vi "WPI_UtilitiesFRCAutomaticValuePublisherImpl.vi"(11 "Enable":bool=TRUE) -> ()   [LabVIEW 2017]
uses:
  <vilib>/Rock Robotics/WPI/Utilities/Refnum Registry Operation.ctl
  <vilib>/Rock Robotics/WPI/Ultrasonic/WPI_SonarSRF04DigitalRefNum Registry Get.vi
  <vilib>/Rock Robotics/WPI/Ultrasonic/WPI_SonarSRF04DigitalGetRange.vi
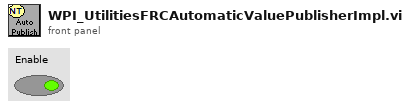
[diagram p1: front panel]
types:
  T1 = typedef "Refnum Registry Operation.ctl" = enum16{"set", "get", "delete", "get all names", "read name"}
  T2 = typedef "WPI_JoystickDevRef.ctl" = cluster{"Device":T3}
  T3 = typedef "WPI_JoystickDeviceEnum.ctl" = enum16{"USB 0", "USB 1", "USB 2", "USB 3", "USB 4", "USB 5"}
  T4 = typedef "WPI_Joystick Info.ctl" = cluster{"Device Name":string, "HID Type":T5, "XBox Type":T6, "Axes Count":i32, "Axes Types":T7[], "Button Count":i32, "POV Count":i32}
  T5 = typedef "WPI_JoystickHID Types.ctl" = enum16{"Not HID", "HID Joystick", "HID Gamepad", "HID Driving Wheel", "HID Flightstick", "HID First Person"}
  T6 = typedef "WPI_JoystickXBox Types.ctl" = enum16{"Not XBox", "XBox Unknown", "XBox Gamepad", "XBox Wheel", "XBox Arcade Stick", "XBox Flight Stick", "XBox Dance Pad", "XBox Guitar", "XBox Drum Kit", "XBox Arcade Pad"}
  T7 = typedef "WPI_JoystickAxis Types.ctl" = enum16{"X Axis", "Y Axis", "Z Axis", "RxAxis", "RyAxis", "RzAxis", "Slider", "POV", "None", "L X Axis", "L Y Axis", "L Trigger", "R Trigger", "R X Axis", "R Y Axis"}
  T8 = typedef "WPI_MotorControlDeviceRef.ctl" = cluster{"DeviceStatus":errorcluster, "Type":T9, "PWM":cluster{"PWM Channel":T10, "DeadBand":T11}, "CAN":cluster{"Device Number":u8, "SetOutput VI Ref":variant, "GetOutput VI Ref":variant, "Enable VI Ref":variant, "Disable VI Ref":variant, "Data":variant}, "Invert":bool, "DIO PWM":cluster{"PWM \"Enable\" Channel":T10, "DIOChannel":T12, "PWM Rate":dbl}}
  T9 = typedef "WPI_MotorControlType.ctl" = enum16{"PWM", "CAN", "DIO PWM"}
  T10 = typedef "FPGA_DIOPWMChannel.ctl" = enum8{"PWM 0", "PWM 1", "PWM 2", "PWM 3", "PWM 4", "PWM 5", "PWM 6", "PWM 7", "PWM 8", "PWM 9", "PWM MXP 0", "PWM MXP 1", "PWM MXP 2", "PWM MXP 3", "PWM MXP 4", "PWM MXP 5", "PWM MXP 6", "PWM MXP 7", "PWM MXP 8", "PWM MXP 9", "Invalid"}
  T11 = typedef "WPI_PWMDeadband.ctl" = cluster{"Name":string, "maxPositivePwm":i32, "minPositivePwm":i32, "centerPwm":i32, "maxNegativePwm":i32, "minNegativePwm":i32, "angularRange":u16}
  T12 = typedef "FPGA_DIOChannel.ctl" = enum8{"DIO 0", "DIO 1", "DIO 2", "DIO 3", "DIO 4", "DIO 5", "DIO 6", "DIO 7", "DIO 8", "DIO 9", "DIO MXP 0", "DIO MXP 1", "DIO MXP 2", "DIO MXP 3", "DIO MXP 4", "DIO MXP 5", "DIO MXP 6", "DIO MXP 7", "DIO MXP 8", "DIO MXP 9", "DIO MXP 10", "DIO MXP 11", "DIO MXP 12", "DIO MXP 13", "DIO MXP 14", "DIO MXP 15", "SPI Port CS1", "SPI Port CS2", "SPI Port CS3", "SPI Port MISO", "SPI Port MOSI", "Invalid"}
  T13 = typedef "WPI_ServoDeviceRef.ctl" = cluster{"DeviceStatus":errorcluster, "PWM Channel":T10, "DeadBand":T11}
  T14 = typedef "WPI_GyroDevRef.ctl" = cluster{"DevStatus":errorcluster, "Analog Channel":T15, "Gain (VoltsPerDegree/Second)":dbl, "Gyro Type":enum16{"Analog", "XRS450"}, "Handle":i32, "SPI Bus":T16, "Device Found":bool, "Sample Rate":dbl, "Calibrate On Open":bool, "Offset":dbl}
  T15 = typedef "FPGA_AIChannel.ctl" = enum8{"AI 0", "AI 1", "AI 2", "AI 3", "AI MXP 0", "AI MXP 1", "AI MXP 2", "AI MXP 3", "Invalid"}
  T16 = typedef "spi_bus.ctl" = enum16{"SPI On-Board, CS0", "SPI On-Board, CS1", "SPI On-Board, CS2", "SPI On-Board, CS3", "SPI MXP", "Invalid"}
  T17 = typedef "WPI_UltrasonicDeviceRef.ctl" = cluster{"DevStatus":errorcluster, "Ping Channel":T12, "Echo Channel":T12, "CntIndex":T18}
  T18 = typedef "FPGA_CounterCtrSystemIndex.ctl" = enum8{"Ctr 0", "Ctr 1", "Ctr 2", "Ctr 3", "Ctr 4", "Ctr 5", "Ctr 6", "Ctr 7", "Invalid"}
  T19 = typedef "WPI_EncoderDevRef.ctl" = cluster{"DevStatus":errorcluster, "EncoderIndex":T20, "CounterIndex":T18, "DistancePerCount":dbl, "Decoding Type":T21}
  T20 = typedef "FPGA_EncoderIdx.ctl" = enum8{"Enc 0", "Enc 1", "Enc 2", "Enc 3", "Enc 4", "Enc 5", "Enc 6", "Enc 7", "Invalid"}
  T21 = typedef "WPI_EncoderType.ctl" = enum16{"1x", "2x", "4x"}
  T22 = typedef "WPI_CameraDevRef.ctl" = cluster{"Camera Address":string, "CameraStatus":errorcluster}
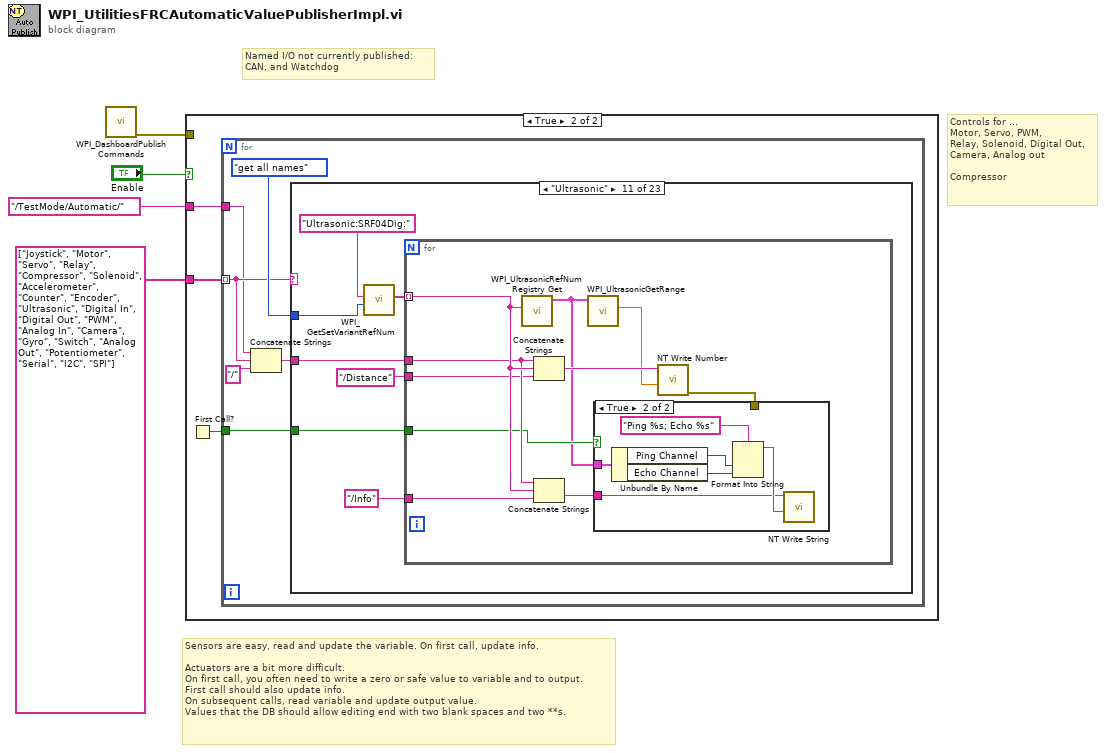
[diagram p0: block diagram]
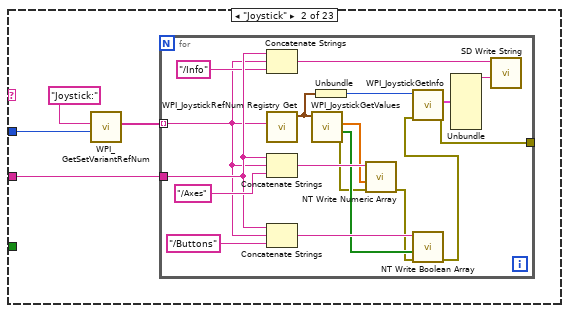
[diagram p4: hidden frame]
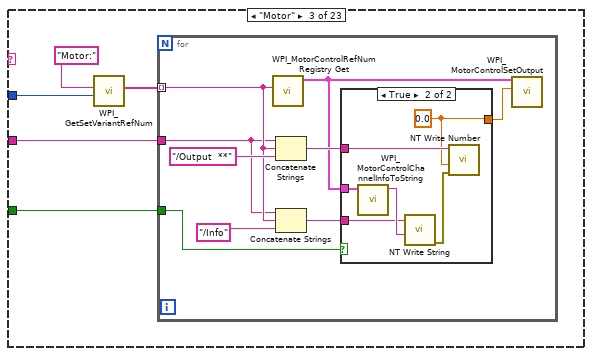
[diagram p5: hidden frame]
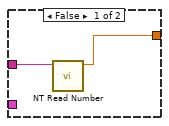
[diagram p6: hidden frame]
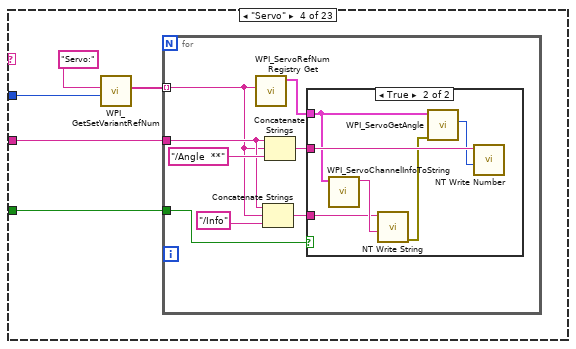
[diagram p7: hidden frame]
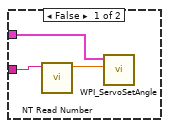
[diagram p8: hidden frame]
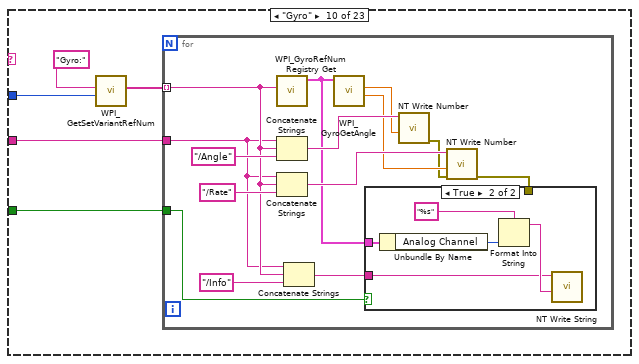
[diagram p14: hidden frame]
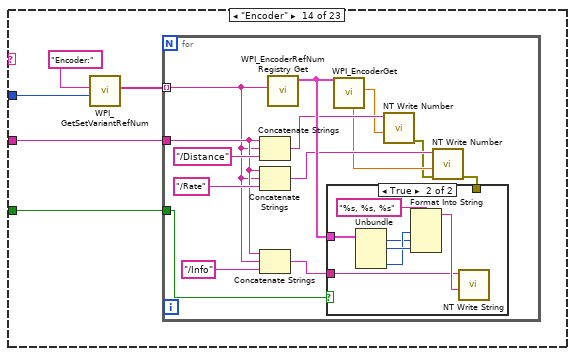
[diagram p19: hidden frame]
diagram:
  # "Controls for ...\nMotor, Servo, PWM,\nRelay, Solenoid, Digital Out,\nCamera, Analog out\n\nCompressor"
  # "Named I/O not currently published:\nCAN, and Watchdog"
  # "Sensors are easy, read and update the variable. On first call, update info.\n\nActuators are a bit more difficult. \nOn first call, you often need to write a zero or safe value to variable and to output.\nFirst call should also update info.\nOn subsequent calls, read variable and update output value.\nValues that the DB should allow editing end with two blank spaces and two **s."
  n1 = call <vilib>:"WPI_DashboardPublish Commands.vi"() -> ("error out"=w1:errorcluster)  [unwired: 11 in]
  n2 = case shown="True" "Enable" {
    tunnel: string[] ["Joystick", "Motor", "Servo", "Relay", "Compressor", "Solenoid", "Accelerometer", "Counter", "Encoder", "Ultrasonic", "Digital In", "Digital Out", "PWM", "Analog In", "Camera", "Gyro", "Switch", "Analog Out", "Potentiometer", "Serial", "I2C", "SPI"] -> [_ w7]
    tunnel: "/TestMode/Automatic/" -> [_ w5]
    tunnel: w1 -> [_ _]
    frame False {
    }
    frame True {
      n3 = First Call?() -> (First Call?: T/F=w6:bool)
      n4 = for {
        tunnel: w7 -> [w11] mode=indexing
        tunnel: w6 -> [w12]
        tunnel: w5 -> [w10]
        n5 = Concatenate Strings(w10, w11, "/") -> (w8:string)
        n6 = case shown="\"Ultrasonic\"" w11 {
          tunnel: Refnum_Registry_Operation."get all names" ("menu") -> [_ w15 w37 w58 _ _ _ _ _ w80 w108 _ _ w127 _ _ _ _ _ w153 _ _ _]
          tunnel: w12 -> [_ _ w40 w62 _ _ _ _ _ w84 w110 _ _ w131 _ _ _ _ _ w157 _ _ _]
          tunnel: w8 -> [_ w17 w39 w61 _ _ _ _ _ w83 w109 _ _ w130 _ _ _ _ _ w156 _ _ _]
          frame Default {
            # "Unsupported I/O type"
          }
          frame "Joystick" {
            n7 = call <vilib>:"WPI_GetSetVariantRefNum.vi"("Operation"=w15, "refnum name"="Joystick:") -> ("names"=w16:string[])  [unwired: 7 in, 2 out]
            n8 = for {
              tunnel: w16 -> [w24] mode=indexing
              tunnel: w17 -> [w26]
              tunnel: [w18] -> _
              n9 = Concatenate Strings(w26, w24, "/Info") -> (w23:string)
              n10 = call <vilib>:"WPI_JoystickRefNum Registry Get.vi"("refnum name"=w24) -> ("JoystickDevRef"=w29:T2)  [unwired: 9 in, 1 out]
              n11 = Concatenate Strings(w26, w24, "/Axes") -> (w32:string)
              n12 = Concatenate Strings(w26, w24, "/Buttons") -> (w34:string)
              n13 = call <vilib>:"WPI_JoystickGetValues.vi"("JoystickDevRef"=w29) -> ("error out"=w19:errorcluster, "Buttons"=w30:bool[], "Axes"=w31:dbl[])  [unwired: 6 in, 2 out]
              n14 = Unbundle(w29) -> ("Device"=w28:T3)
              n15 = call <vilib>:"NT Write Numeric Array.vi"("error in"=w19, "Numeric Array"=w31, "Name"=w32) -> ("error out"=w21:errorcluster)  [unwired: 8 in]
              n16 = call <vilib>:"NT Write Boolean Array.vi"("error in"=w21, "Boolean Array"=w30, "Name"=w34) -> ("error out"=w20:errorcluster)  [unwired: 8 in]
              n17 = call <vilib>:"WPI_JoystickGetInfo.vi"("error in (no error)"=w20, "JoystickDevice"=w28) -> ("error out"=w18:errorcluster, "Joystick Info"=w27:T4)  [unwired: 8 in]
              n18 = Unbundle(w27) -> ("Device Name"=w22:string)  [unwired: 6 out]
              n19 = call <vilib>:"SD Write String.vi"("String"=w22, "Name"=w23) -> ()  [unwired: 8 in, 2 out]
            }
          }
          frame "Motor" {
            n20 = call <vilib>:"WPI_GetSetVariantRefNum.vi"("Operation"=w37, "refnum name"="Motor:") -> ("names"=w36:string[])  [unwired: 7 in, 2 out]
            n21 = for {
              tunnel: w36 -> [w44] mode=indexing
              tunnel: w40 -> [w46]
              tunnel: w39 -> [w43]
              n22 = call <vilib>:"WPI_MotorControlRefNum Registry Get.vi"("refnum name"=w44) -> ("MotorControlDevRef"=w42:T8)  [unwired: 9 in, 1 out]
              n23 = Concatenate Strings(w43, w44, "/Output  **") -> (w48:string)
              n24 = Concatenate Strings(w43, w44, "/Info") -> (w41:string)
              n25 = case shown="True" w46 {
                tunnel: w48 -> [w51 w57]
                tunnel: [w50 w56] -> w47
                tunnel: w42 -> [_ w54]
                tunnel: w41 -> [_ w53]
                frame False {
                  n26 = call <vilib>:"NT Read Number.vi"("Name"=w51) -> ("Numeric"=w50:dbl)  [unwired: 9 in, 1 out]
                }
                frame True {
                  w56 = 0.0
                  n27 = call <vilib>:"WPI_MotorControlChannelInfoToString.vi"("MotorControlDevRef"=w54) -> ("String"=w55:string)  [unwired: 10 in]
                  n28 = call <vilib>:"NT Write String.vi"("String"=w55, "Name"=w53) -> ("error out"=w52:errorcluster)  [unwired: 9 in]
                  n29 = call <vilib>:"NT Write Number.vi"("error in"=w52, "Numeric"=w56, "Name"=w57) -> ()  [unwired: 8 in, 1 out]
                }
              }
              n30 = call <vilib>:"WPI_MotorControlSetOutput.vi"("Output"=w47, "MotorControlDevRef"=w42) -> ()  [unwired: 7 in, 3 out]
            }
          }
          frame "Servo" {
            n31 = call <vilib>:"WPI_GetSetVariantRefNum.vi"("Operation"=w58, "refnum name"="Servo:") -> ("names"=w59:string[])  [unwired: 7 in, 2 out]
            n32 = for {
              tunnel: w59 -> [w63] mode=indexing
              tunnel: w62 -> [w68]
              tunnel: w61 -> [w65]
              n33 = call <vilib>:"WPI_ServoRefNum Registry Get.vi"("refnum name"=w63) -> ("ServoDeviceRef"=w67:T13)  [unwired: 9 in, 1 out]
              n34 = Concatenate Strings(w65, w63, "/Info") -> (w64:string)
              n35 = Concatenate Strings(w65, w63, "/Angle  **") -> (w69:string)
              n36 = case shown="True" w68 {
                tunnel: w69 -> [w73 w79]
                tunnel: w67 -> [w71 w77]
                tunnel: w64 -> [_ w75]
                frame False {
                  n37 = call <vilib>:"NT Read Number.vi"("Name"=w73) -> ("Numeric"=w72:dbl)  [unwired: 9 in, 1 out]
                  n38 = call <vilib>:"WPI_ServoSetAngle.vi"("Angle"=w72, "ServoDeviceRef"=w71) -> ()  [unwired: 8 in, 2 out]
                }
                frame True {
                  n39 = call <vilib>:"WPI_ServoChannelInfoToString.vi"("ServoDeviceRef"=w77) -> ("String"=w76:string)  [unwired: 10 in]
                  n40 = call <vilib>:"NT Write String.vi"("String"=w76, "Name"=w75) -> ("error out"=w74:errorcluster)  [unwired: 9 in]
                  n41 = call <vilib>:"WPI_ServoGetAngle.vi"("ServoDeviceRef"=w77, "error in (no error)"=w74) -> ("Angle"=w78:u16)  [unwired: 6 in, 2 out]
                  n42 = call <vilib>:"NT Write Number.vi"("Numeric"=w78, "Name"=w79) -> ()  [unwired: 9 in, 1 out]
                }
              }
            }
          }
          frame "Relay" {
            # "Not supported in simulation"
          }
          frame "Compressor" {
            # "Not supported in simulation"
          }
          frame "Solenoid" {
            # "Not supported in simulation"
          }
          frame "Accelerometer" {
            # "Not supported in simulation"
          }
          frame "Counter" {
            # "Not supported in simulation"
          }
          frame "Gyro" {
            n43 = call <vilib>:"WPI_GetSetVariantRefNum.vi"("Operation"=w80, "refnum name"="Gyro:") -> ("names"=w81:string[])  [unwired: 7 in, 2 out]
            n44 = for {
              tunnel: w81 -> [w91] mode=indexing
              tunnel: w84 -> [w88]
              tunnel: w83 -> [w90]
              n45 = call <vilib>:"WPI_GyroRefNum Registry Get.vi"("refnum name"=w91) -> ("GyroDevRef"=w87:T14)  [unwired: 9 in, 1 out]
              n46 = Concatenate Strings(w90, w91, "/Angle") -> (w97:string)
              n47 = Concatenate Strings(w90, w91, "/Rate") -> (w95:string)
              n48 = Concatenate Strings(w90, w91, "/Info") -> (w89:string)
              n49 = call <vilib>:"WPI_GyroGetAngle.vi"("GyroDevRef"=w87) -> ("Angular Rate"=w93:dbl, "Angle"=w94:dbl)  [unwired: 6 in, 3 out]
              n50 = call <vilib>:"NT Write Number.vi"("Numeric"=w94, "Name"=w97) -> ("error out"=w86:errorcluster)  [unwired: 9 in]
              n51 = call <vilib>:"NT Write Number.vi"("error in"=w86, "Numeric"=w93, "Name"=w95) -> ("error out"=w85:errorcluster)  [unwired: 8 in]
              n52 = case shown="True" w88 {
                tunnel: w89 -> [_ w101]
                tunnel: w87 -> [_ w100]
                tunnel: w85 -> [_ _]
                frame False {
                }
                frame True {
                  n53 = Unbundle By Name(w100) -> ("Analog Channel"=w99:T15)
                  n54 = Format Into String(format string="%s", w99) -> (resulting string=w102:string)  [unwired: 2 in, 1 out]
                  n55 = call <vilib>:"NT Write String.vi"("String"=w102, "Name"=w101) -> ()  [unwired: 9 in, 1 out]
                }
              }
            }
          }
          frame "Ultrasonic" {
            n56 = call <vilib>:"WPI_GetSetVariantRefNum.vi"("Operation"=w108, "refnum name"="Ultrasonic:SRF04Dig:") -> ("names"=w107:string[])  [unwired: 7 in, 2 out]
            n57 = for {
              tunnel: w107 -> [w120] mode=indexing
              tunnel: w110 -> [w118]
              tunnel: w109 -> [w119]
              tunnel: "/Info" -> [w117]
              tunnel: "/Distance" -> [w116]
              n58 = call-poly <vilib>:"WPI_UltrasonicRefNum Registry Get.vi"("refnum name"=w120) -> ("SonarSRF04DevRef"=w112:T17)  [unwired: 9 in, 1 out]
              n59 = Concatenate Strings(w119, w120, w116) -> (w115:string)
              n60 = Concatenate Strings(w119, w120, w117) -> (w113:string)
              n61 = call-poly <vilib>:"WPI_UltrasonicGetRange.vi"("SonarSRF04DevRef"=w112) -> ("Distance"=w114:dbl)  [unwired: 8 in, 2 out]
              n62 = call <vilib>:"NT Write Number.vi"("Numeric"=w114, "Name"=w115) -> ("error out"=w111:errorcluster)  [unwired: 9 in]
              n63 = case shown="True" w118 {
                tunnel: w113 -> [_ w125]
                tunnel: w112 -> [_ w124]
                tunnel: w111 -> [_ _]
                frame False {
                }
                frame True {
                  n64 = Unbundle By Name(w124) -> ("Ping Channel"=w123:T12, "Echo Channel"=w122:T12)
                  n65 = Format Into String(format string="Ping %s; Echo %s", w123, w122) -> (resulting string=w126:string)  [unwired: 2 in, 1 out]
                  n66 = call <vilib>:"NT Write String.vi"("String"=w126, "Name"=w125) -> ()  [unwired: 9 in, 1 out]
                }
              }
            }
          }
          frame "Digital In" {
            # "Not supported in simulation"
          }
          frame "Switch" {
            # "Not supported in simulation"
          }
          frame "Encoder" {
            n67 = call <vilib>:"WPI_GetSetVariantRefNum.vi"("Operation"=w127, "refnum name"="Encoder:") -> ("names"=w128:string[])  [unwired: 7 in, 2 out]
            n68 = for {
              tunnel: w128 -> [w134] mode=indexing
              tunnel: w131 -> [w143]
              tunnel: w130 -> [w135]
              n69 = Concatenate Strings(w135, w134, "/Distance") -> (w140:string)
              n70 = Concatenate Strings(w135, w134, "/Rate") -> (w137:string)
              n71 = Concatenate Strings(w135, w134, "/Info") -> (w142:string)
              n72 = call <vilib>:"WPI_EncoderRefNum Registry Get.vi"("refnum name"=w134) -> ("EncoderDevRef"=w141:T19)  [unwired: 9 in, 1 out]
              n73 = call <vilib>:"WPI_EncoderGet.vi"("EncoderDevRef"=w141) -> ("Distance"=w139:dbl, "Rate"=w136:dbl)  [unwired: 5 in, 4 out]
              n74 = call <vilib>:"NT Write Number.vi"("Numeric"=w139, "Name"=w140) -> ("error out"=w133:errorcluster)  [unwired: 9 in]
              n75 = call <vilib>:"NT Write Number.vi"("error in"=w133, "Numeric"=w136, "Name"=w137) -> ("error out"=w132:errorcluster)  [unwired: 8 in]
              n76 = case shown="True" w143 {
                tunnel: w142 -> [_ w149]
                tunnel: w141 -> [_ w146]
                tunnel: w132 -> [_ _]
                frame False {
                }
                frame True {
                  n77 = Unbundle(w146) -> ("EncoderIndex"=w147:T20, "CounterIndex"=w152:T18, "Decoding Type"=w148:T21)  [unwired: 2 out]
                  n78 = Format Into String(format string="%s, %s, %s", w148, w147, w152) -> (resulting string=w150:string)  [unwired: 2 in, 1 out]
                  n79 = call <vilib>:"NT Write String.vi"("String"=w150, "Name"=w149) -> ()  [unwired: 9 in, 1 out]
                }
              }
            }
          }
          frame "Digital Out" {
            # "Not supported in simulation"
          }
          frame "Analog Out" {
            # "Not supported in simulation"
          }
          frame "PWM" {
            # "Not supported in simulation"
          }
          frame "Analog In" {
            # "Not supported in simulation"
          }
          frame "Potentiometer" {
            # "Not supported in simulation"
          }
          frame "Camera" {
            n80 = call <vilib>:"WPI_GetSetVariantRefNum.vi"("Operation"=w153, "refnum name"="Camera:") -> ("names"=w154:string[])  [unwired: 7 in, 2 out]
            n81 = for {
              tunnel: w154 -> [w161] mode=indexing
              tunnel: w157 -> [w163]
              tunnel: w156 -> [w162]
              n82 = call <vilib>:"WPI_CameraRefNum Registry Get.vi"("refnum name"=w161) -> ("CameraDevRef"=w160:T22)  [unwired: 9 in, 1 out]
              n83 = Unbundle By Name(w160) -> ("Camera Address"=w159:string)
              n84 = call <vilib>:"WPI_CameraIsSimulated.vi"("Camera Address"=w159) -> ("Simulated"=w158:bool)  [unwired: 10 in]
              n85 = case shown="False" w158 {
                tunnel: w163 -> [w167 _]
                tunnel: w162 -> [w166 _]
                tunnel: w161 -> [w165 _]
                tunnel: w160 -> [w164 _]
                frame False {
                  n86 = case shown="True" w167 {
                    tunnel: w164 -> [w170 w173]
                    tunnel: w166 -> [w169 w172]
                    tunnel: w165 -> [w168 w171]
                    frame False {
                      n87 = call <vilib>:"WPI_CameraUpdate Settings.vi"("Name"=w168, "Table"=w169, "CameraDevRef"=w170) -> ()  [unwired: 9 in]
                    }
                    frame True {
                      n88 = call <vilib>:"WPI_CameraPublish Settings.vi"("Name"=w171, "Table"=w172, "CameraDevRef"=w173) -> ()  [unwired: 9 in]
                    }
                  }
                }
                frame True {
                  # "ignore for simulation"
                }
              }
            }
          }
          frame "Serial" {
            # "Not supported in simulation"
          }
          frame "I2C" {
            # "Not supported in simulation"
          }
          frame "SPI" {
            # "Not supported in simulation"
          }
        }
      }
    }
  }
